vi "SubVI_TurnL3ft_Auto.vi"(8 "Speed":dbl=1000.0, 9 "degrees to turn left":dbl=90.0 format="%#_13g") -> ()   [LabVIEW 2017]
uses:
  <vilib>/Rock Robotics/WPI/ThirdParty/Sensors/navX/_TypeDefs/Z900_navX_ActionTypeDef.ctl
  <vilib>/Rock Robotics/WPI/ThirdParty/Sensors/navX/_TypeDefs/FRIC_navX_DeviceNumbersTypeDef.ctl
  <vilib>/Rock Robotics/WPI/ThirdParty/Phoenix-LabVIEW/Motor Controller/Controls/CTRE_Phoenix_MotorControl_ControlMode.ctl
  <vilib>/Rock Robotics/WPI/ThirdParty/Phoenix-LabVIEW/Pigeon IMU/CTRE_PigeonIMU_GetYPR.vi
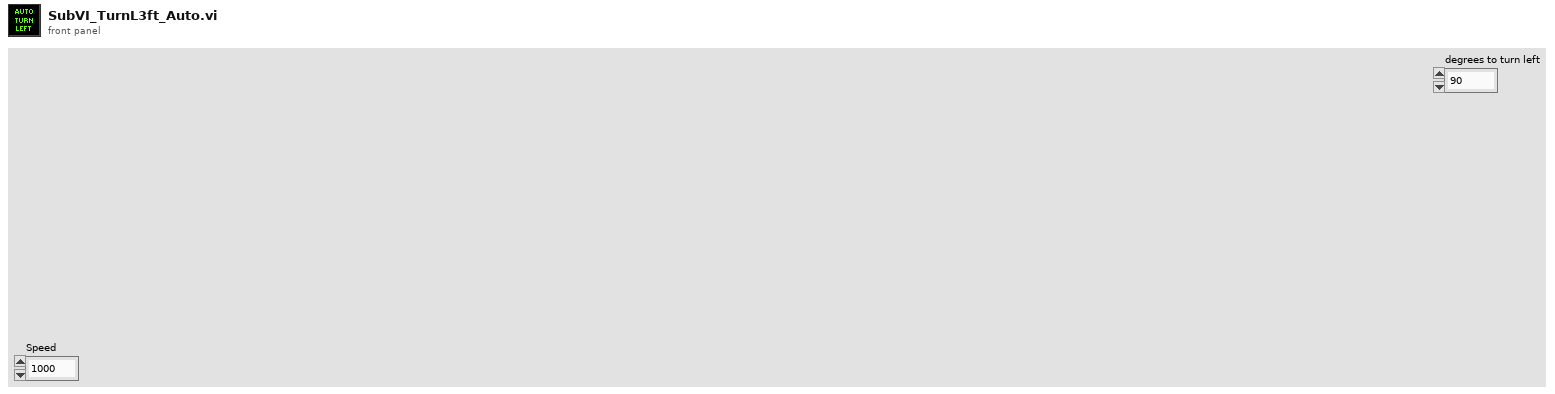
[diagram p1: front panel]
types:
  T1 = typedef "FRIC_navX_DeviceNumbersTypeDef.ctl" = enum16{"Dev0", "Dev1", "Dev2", "Dev3"}
  T2 = typedef "Z900_navX_ActionTypeDef.ctl" = enum16{"None", "Halt", "Normal Read", "Update Serial Protocol", "Update Rate Htz", "Zero-Yaw", "Zero-Displacement", "Zero-Velocity"}
  T3 = typedef "WPI_MotorControlDeviceRef.ctl" = cluster{"DeviceStatus":errorcluster, "Type":T4, "PWM":cluster{"PWM Channel":T5, "DeadBand":T6}, "CAN":cluster{"Device Number":u8, "SetOutput VI Ref":variant, "GetOutput VI Ref":variant, "Enable VI Ref":variant, "Disable VI Ref":variant, "Data":variant}, "Invert":bool, "DIO PWM":cluster{"PWM \"Enable\" Channel":T5, "DIOChannel":T7, "PWM Rate":dbl}}
  T4 = typedef "WPI_MotorControlType.ctl" = enum16{"PWM", "CAN", "DIO PWM"}
  T5 = typedef "FPGA_DIOPWMChannel.ctl" = enum8{"PWM 0", "PWM 1", "PWM 2", "PWM 3", "PWM 4", "PWM 5", "PWM 6", "PWM 7", "PWM 8", "PWM 9", "PWM MXP 0", "PWM MXP 1", "PWM MXP 2", "PWM MXP 3", "PWM MXP 4", "PWM MXP 5", "PWM MXP 6", "PWM MXP 7", "PWM MXP 8", "PWM MXP 9", "Invalid"}
  T6 = typedef "WPI_PWMDeadband.ctl" = cluster{"Name":string, "maxPositivePwm":i32, "minPositivePwm":i32, "centerPwm":i32, "maxNegativePwm":i32, "minNegativePwm":i32, "angularRange":u16}
  T7 = typedef "FPGA_DIOChannel.ctl" = enum8{"DIO 0", "DIO 1", "DIO 2", "DIO 3", "DIO 4", "DIO 5", "DIO 6", "DIO 7", "DIO 8", "DIO 9", "DIO MXP 0", "DIO MXP 1", "DIO MXP 2", "DIO MXP 3", "DIO MXP 4", "DIO MXP 5", "DIO MXP 6", "DIO MXP 7", "DIO MXP 8", "DIO MXP 9", "DIO MXP 10", "DIO MXP 11", "DIO MXP 12", "DIO MXP 13", "DIO MXP 14", "DIO MXP 15", "SPI Port CS1", "SPI Port CS2", "SPI Port CS3", "SPI Port MISO", "SPI Port MOSI", "Invalid"}
  T8 = typedef "CTRE_PigeonIMU_DeviceRef.ctl" = cluster{"DeviceStatus":errorcluster, "Device Number":u8, "Type":T9, "Device ID":u32, "Handle":u64, "UsageFrame":u32, "Library Path":path}
  T9 = typedef "CTRE_PigeonIMU_ConnectionType.ctl" = u32
  T10 = typedef "CTRE_Phoenix_MotorControl_ControlMode.ctl" = u16
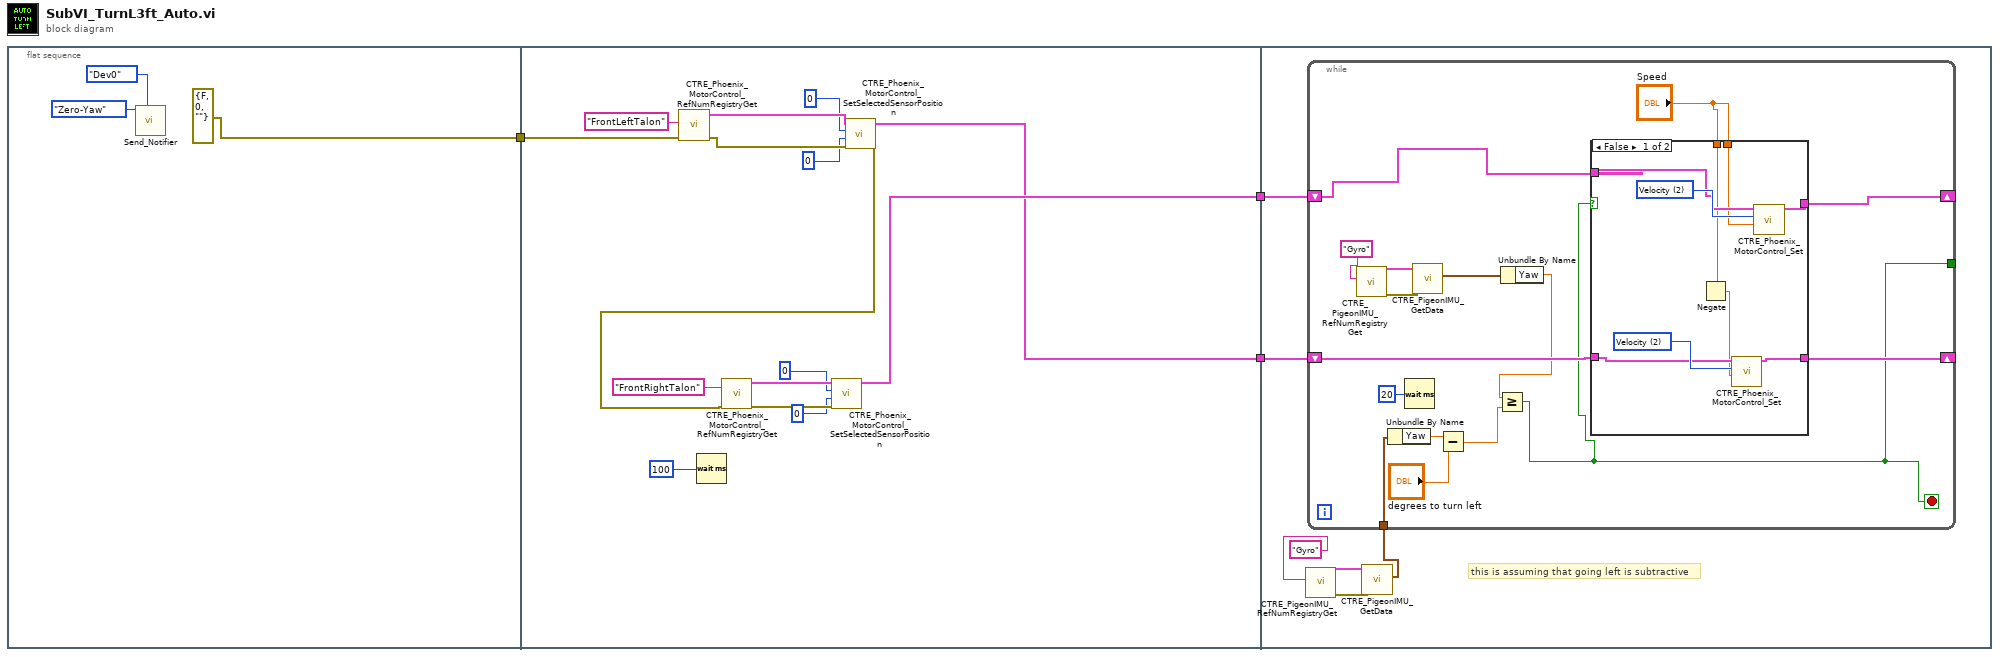
[diagram p0: block diagram]
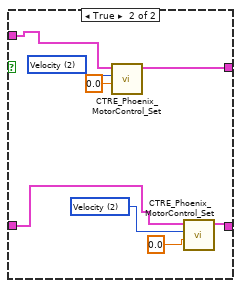
[diagram p2: hidden frame]
diagram:
  n1 = flat-sequence {
    tunnel: [errorcluster {"status"=FALSE, "code"=0, "source"=""} ("error constant")] -> w1
    tunnel: [w9] -> w3
    tunnel: [w8] -> w2
    tunnel: w1 -> [w11]
    tunnel: w3 -> [w27]
    tunnel: w2 -> [w26]
    frame #0 {
      n2 = call <vilib>:"Send_Notifier.vi"("Device Number"=FRIC_navX_DeviceNumbersTypeDef."Dev0", "navX Action"=Z900_navX_ActionTypeDef."Zero-Yaw") -> ()  [unwired: 10 in]
    }
    frame #1 {
      n3 = call <vilib>:"CTRE_Phoenix_MotorControl_RefNumRegistryGet.vi"("error in (no error)"=w11, "refnum name"="FrontLeftTalon") -> ("error out"=w18:errorcluster, "PhoenixMotorControlDevRef"=w20:T3)  [unwired: 8 in]
      n4 = Wait (ms)(milliseconds to wait=u32 100) -> ()  [unwired: 1 out]
      n5 = call <vilib>:"CTRE_Phoenix_MotorControl_SetSelectedSensorPosition.vi"("error in (no error)"=w18, "pidLoopIdx"=0 ("New Sensor Position"), "New Sensor Position"=u32 0 ("pidLoopIdx"), "PhoenixMotorControlDevRef"=w20) -> ("error out"=w7:errorcluster, "PhoenixMotorControlDevRef"=w8:T3)  [unwired: 6 in]
      n6 = call <vilib>:"CTRE_Phoenix_MotorControl_RefNumRegistryGet.vi"("error in (no error)"=w7, "refnum name"="FrontRightTalon") -> ("error out"=w17:errorcluster, "PhoenixMotorControlDevRef"=w19:T3)  [unwired: 8 in]
      n7 = call <vilib>:"CTRE_Phoenix_MotorControl_SetSelectedSensorPosition.vi"("error in (no error)"=w17, "pidLoopIdx"=0 ("New Sensor Position"), "New Sensor Position"=u32 0 ("pidLoopIdx"), "PhoenixMotorControlDevRef"=w19) -> ("PhoenixMotorControlDevRef"=w9:T3)  [unwired: 6 in, 1 out]
    }
    frame #2 {
      # "this is assuming that going left is subtractive"
      n8 = call <vilib>:"CTRE_PigeonIMU_RefNumRegistryGet.vi"("refnum name"="Gyro") -> ("error out"=w25:errorcluster, "PigeonIMUDevRef"=w24:T8)  [unwired: 9 in]
      n9 = call-poly <vilib>:"CTRE_PigeonIMU_GetData.vi"("error in (no error)"=w25, "PigeonIMUDevRef"=w24) -> ("Yaw Pitch Roll"=w22:cluster{"Yaw":dbl, "Pitch":dbl, "Roll":dbl})  [unwired: 7 in, 2 out]
      n10 = while {
        shift-right: [w40] -> _
        shift-left: w26 -> [w41]
        shift-right: [w43] -> _
        shift-left: w27 -> [w42]
        tunnel: [w33] -> _
        tunnel: w22 -> [w34]
        stop <- w33 stop-if-true
        n11 = call <vilib>:"CTRE_PigeonIMU_RefNumRegistryGet.vi"("refnum name"="Gyro") -> ("error out"=w31:errorcluster, "PigeonIMUDevRef"=w32:T8)  [unwired: 9 in]
        n12 = Unbundle By Name(w34) -> ("Yaw"=w37:dbl)
        n13 = Wait (ms)(milliseconds to wait=u32 20) -> ()  [unwired: 1 out]
        n14 = call-poly <vilib>:"CTRE_PigeonIMU_GetData.vi"("error in (no error)"=w31, "PigeonIMUDevRef"=w32) -> ("Yaw Pitch Roll"=w29:cluster{"Yaw":dbl, "Pitch":dbl, "Roll":dbl})  [unwired: 7 in, 2 out]
        n15 = Subtract(x=w37, y="degrees to turn left") -> (x-y=w35:dbl)
        n16 = Unbundle By Name(w29) -> ("Yaw"=w28:dbl)
        n17 = Greater Or Equal?(x=w28, y=w35) -> (x >= y?=w33:bool)
        n18 = case shown="False" w33 {
          tunnel: [w51 w58] -> w43
          tunnel: w42 -> [w50 w57]
          tunnel: w41 -> [w48 w55]
          tunnel: [w47 w53] -> w40
          tunnel: "Speed" -> [w46 _]
          tunnel: "Speed" -> [w45 _]
          frame False {
            w49 = T10 2 items=["PercentOutput"=0, "Position"=1, "Velocity"=2, "Current"=3, "Follower"=5, "MotionProfile"=6, "MotionMagic"=7, "MotionMagicArc"=8, "MotionProfileArc"=10, "Disabled"=15] ("Control Mode")
            w52 = T10 2 items=["PercentOutput"=0, "Position"=1, "Velocity"=2, "Current"=3, "Follower"=5, "MotionProfile"=6, "MotionMagic"=7, "MotionMagicArc"=8, "MotionProfileArc"=10, "Disabled"=15] ("Control Mode")
            n19 = Negate(x=w45) -> (-x=w44:dbl)
            n20 = call <vilib>:"CTRE_Phoenix_MotorControl_Set.vi"("Output"=w44, "Control Mode"=w49, "PhoenixMotorControlDevRef"=w48) -> ("PhoenixMotorControlDevRef"=w47:T3)  [unwired: 7 in, 1 out]
            n21 = call <vilib>:"CTRE_Phoenix_MotorControl_Set.vi"("Output"=w46, "Control Mode"=w52, "PhoenixMotorControlDevRef"=w50) -> ("PhoenixMotorControlDevRef"=w51:T3)  [unwired: 7 in, 1 out]
          }
          frame True {
            w56 = T10 2 items=["PercentOutput"=0, "Position"=1, "Velocity"=2, "Current"=3, "Follower"=5, "MotionProfile"=6, "MotionMagic"=7, "MotionMagicArc"=8, "MotionProfileArc"=10, "Disabled"=15] ("Control Mode")
            w59 = T10 2 items=["PercentOutput"=0, "Position"=1, "Velocity"=2, "Current"=3, "Follower"=5, "MotionProfile"=6, "MotionMagic"=7, "MotionMagicArc"=8, "MotionProfileArc"=10, "Disabled"=15] ("Control Mode")
            n22 = call <vilib>:"CTRE_Phoenix_MotorControl_Set.vi"("Output"=0.0, "Control Mode"=w59, "PhoenixMotorControlDevRef"=w57) -> ("PhoenixMotorControlDevRef"=w58:T3)  [unwired: 7 in, 1 out]
            n23 = call <vilib>:"CTRE_Phoenix_MotorControl_Set.vi"("Output"=0.0, "Control Mode"=w56, "PhoenixMotorControlDevRef"=w55) -> ("PhoenixMotorControlDevRef"=w53:T3)  [unwired: 7 in, 1 out]
          }
        }
      }
    }
  }
